vi "ValidateInput.vi"(8 "error in (no error)":errorcluster, 10 "Input":string, 11 "EAN-13 in":refnum<class "EAN-13.lvclass">) -> (0 "error out":errorcluster, 2 "OK":bool=TRUE, 3 "EAN-13 out":refnum<class "EAN-13.lvclass">)   [LabVIEW 2013, in "BarCodes.lvlib" / "EAN-13.lvclass"]
doc: "Returns whether the specified input can be expressed in this barcode format. For EAN-13, this is whether the text has 12 characters and they're all digits."
uses:
  EAN-13.lvclass
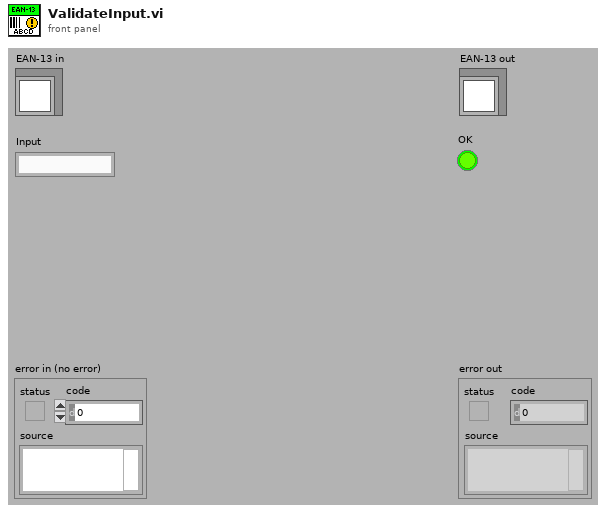
[diagram p1: front panel]
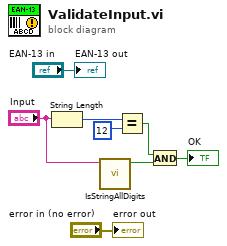
[diagram p0: block diagram]
diagram:
  n1 = String Length(string="Input") -> (length=w1:i32)
  n2 = call "IsStringAllDigits.vi"("String"="Input") -> ("Boolean"=w3:bool)  [unwired: 10 in]
  n3 = Equal?(x=w1, y=12) -> (x = y?=w7:bool)
  n4 = And(x=w7, y=w3) -> (x .and. y?=→"OK":bool)
  "error out" <- "error in (no error)"
  "EAN-13 out" <- "EAN-13 in"
